vi "drawLabel.vi"(0 "reference":refnum<class "StateTransitionEdge.lvclass">, 1 "graphics":refnum<class "Graphics.lvclass">, 5 "error in (no error)":errorcluster) -> (14 "reference out":refnum<class "StateTransitionEdge.lvclass">, 19 "error out":errorcluster)   [LabVIEW 2012, in "StateTransitionEdge.lvclass"]
doc: "private void drawLabel(Graphics2D g2)"
uses:
  <resource>/Framework/Providers/Open_GDS/UML/StateTransitionEdge_class/StateTransitionEdge.lvclass
  <resource>/Framework/Providers/Open_GDS/UML/Graphics_class/Graphics.lvclass
  <resource>/Framework/Providers/Open_GDS/UML/General/Point/Point Point2D.ctl
  <resource>/Framework/Providers/Open_GDS/UML/SegmentedLineEdge_class/SegmentedLineEdge.lvclass
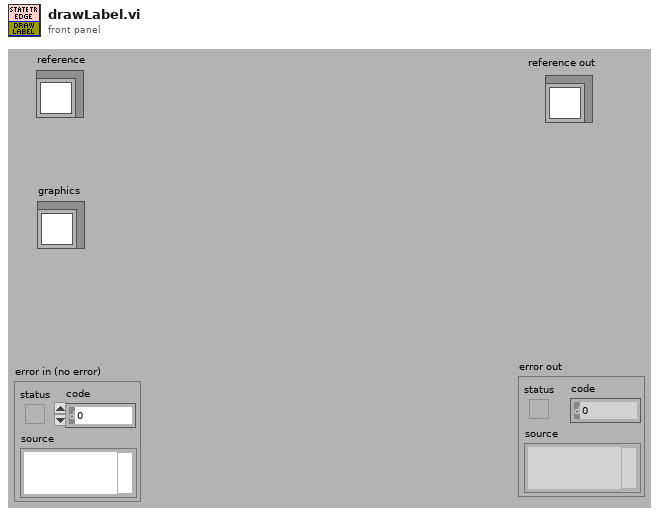
[diagram p1: front panel]
types:
  T1 = typedef "Point Point2D.ctl" = cluster{"x":dbl, "y":dbl}
  T2 = typedef "SegmentedLineEdge.lvclass/ObjectAttributes.ctl" = cluster{"lineStyle":refnum<class "LineStyle.lvclass">, "startArrowHead":refnum<class "ArrowHead.lvclass">, "endArrowHead":refnum<class "ArrowHead.lvclass">, "startLabel":string, "midLabel":string, "endLabel":string, "MidLabelOffset":T1, "SplitWire":bool}
  T3 = typedef "Rectangle Rectangle2D.ctl" = cluster{"x":dbl, "y":dbl, "width":dbl, "height":dbl}
  T4 = cluster{"x":i32, "y":i32, "width":i32, "height":i32}
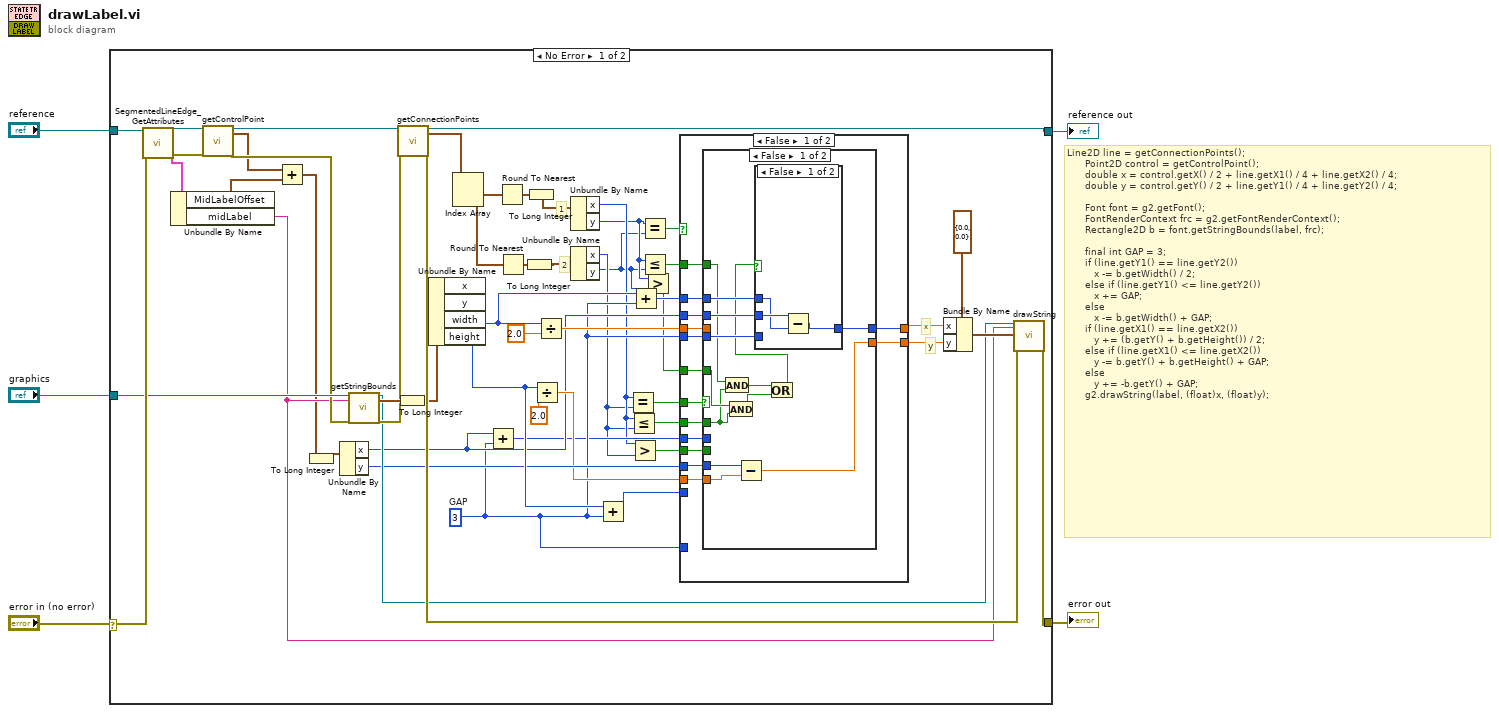
[diagram p0: block diagram]
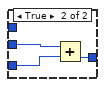
[diagram p2: hidden frame]
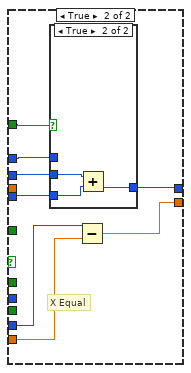
[diagram p3: hidden frame]
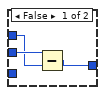
[diagram p4: hidden frame]
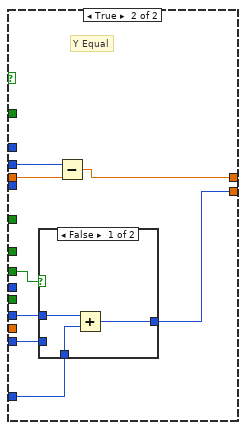
[diagram p5: hidden frame]
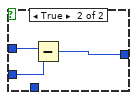
[diagram p6: hidden frame]
diagram:
  # "Line2D line = getConnectionPoints();\n      Point2D control = getControlPoint();\n      double x = control.getX() / 2 + line.getX1() / 4 + line.getX2() / 4;\n      double y = control.getY() / 2 + line.getY1() / 4 + line.getY2() / 4;\n\n      Font font = g2.getFont();\n      FontRenderContext frc = g2.getFontRenderContext();\n      Rectangle2D b = font.getStringBounds(label, frc);      \n\n      final int GAP = 3;\n      if (line.getY1() == line.getY2())\n         x -= b.getWidth() / 2;\n      else if (line.getY1() <= line.getY2())\n         x += GAP;\n      else\n         x -= b.getWidth() + GAP;\n      if (line.getX1() == line.getX2())\n         y += (b.getY() + b.getHeight()) / 2;\n      else if (line.getX1() <= line.getX2())\n         y -= b.getY() + b.getHeight() + GAP;\n      else\n         y += -b.getY() + GAP;\n      g2.drawString(label, (float)x, (float)y);"
  n1 = case shown="No Error" "error in (no error)" {
    selector: "error in (no error)" -> [w57 w120]
    tunnel: "reference" -> [w58 w121]
    tunnel: [w35 w120] -> w4
    tunnel: [w31 w121] -> w3
    tunnel: "graphics" -> [w54 _]
    frame No Error {
      w14 = 3  # GAP
      # "y"
      # "x"
      # "2"
      # "1"
      n2 = call <resource>:"SegmentedLineEdge_GetAttributes.vi"("reference in"=w58, "error in (no error)"=w57) -> ("reference out"=w56:refnum<class "StateTransitionEdge.lvclass">, "Data"=w6:T2, "error out"=w55:errorcluster)  [unwired: 14 in, 1 out]
      n3 = Unbundle By Name(w6) -> ("MidLabelOffset"=w29:T1, "midLabel"=w32:string)
      n4 = call <resource>:"getControlPoint.vi"("reference"=w56, "error in (no error)"=w55) -> ("reference out"=w43:refnum<class "StateTransitionEdge.lvclass">, "point"=w46:T1, "error out"=w53:errorcluster)  [unwired: 15 out]
      n5 = Add(x=w46, y=w29) -> (x+y=w30:T1)
      n6 = To Long Integer(number=w30) -> (32bit integer=w23:cluster{"x":i32, "y":i32})
      n7 = Unbundle By Name(w23) -> ("x"=w15:i32, "y"=w19:i32)
      n8 = call-dynamic "getStringBounds.vi"("reference"=w54, "text"=w32, "error in (no error)"=w53) -> ("reference out"=w33:refnum<class "Graphics.lvclass">, "bounds"=w52:T3, "error out"=w44:errorcluster)  [unwired: 14 in]
      n9 = To Long Integer(number=w52) -> (32bit integer=w24:T4)
      n10 = call-dynamic "getConnectionPoints.vi"("reference"=w43, "error in (no error)"=w44) -> ("reference out"=w31:refnum<class "StateTransitionEdge.lvclass">, "line"=w45:T1[], "error out"=w34:errorcluster)  [unwired: 15 in]
      n11 = Unbundle By Name(w24) -> ("width"=w37:i32, "height"=w22:i32)  [unwired: 2 out]
      n12 = Index Array(array=w45) -> (element #1=w42:T1, element #2=w41:T1)  [unwired: 2 in]
      n13 = Add(x=w15, y=w14) -> (x+y=w13:i32)
      n14 = Round To Nearest(number=w42) -> (nearest integer value=w26:T1)
      n15 = Round To Nearest(number=w41) -> (nearest integer value=w25:T1)
      n16 = To Long Integer(number=w25) -> (32bit integer=w27:cluster{"x":i32, "y":i32})
      n17 = To Long Integer(number=w26) -> (32bit integer=w28:cluster{"x":i32, "y":i32})
      n18 = Divide(x=w22, y=2.0) -> (x/y=w16:dbl)
      n19 = Divide(x=w37, y=2.0) -> (x/y=w40:dbl)
      n20 = Unbundle By Name(w28) -> ("x"=w12:i32, "y"=w10:i32)
      n21 = Unbundle By Name(w27) -> ("x"=w11:i32, "y"=w9:i32)
      n22 = Add(x=w22, y=w14) -> (x+y=w18:i32)
      n23 = Equal?(x=w12, y=w11) -> (x = y?=w17:bool)
      n24 = Less Or Equal?(x=w12, y=w11) -> (x <= y?=w20:bool)
      n25 = Greater?(x=w12, y=w11) -> (0:w7:bool)
      n26 = Add(x=w37, y=w14) -> (x+y=w36:i32)
      n27 = Equal?(x=w10, y=w9) -> (x = y?=w50:bool)
      n28 = Less Or Equal?(x=w10, y=w9) -> (x <= y?=w38:bool)
      n29 = Greater?(x=w10, y=w9) -> (0:w8:bool)
      n30 = case shown="False" w50 {
        tunnel: [w69 w111] -> w48
        tunnel: w15 -> [w71 w113]
        tunnel: w40 -> [w65 w112]
        tunnel: w38 -> [w72 _]
        tunnel: w14 -> [w70 _]
        tunnel: w36 -> [w68 _]
        tunnel: [w66 w107] -> w21
        tunnel: w20 -> [w61 w110]
        tunnel: w19 -> [w64 w109]
        tunnel: w18 -> [_ w108]
        tunnel: w14 -> [_ w106]
        tunnel: w17 -> [w67 _]
        tunnel: w16 -> [w63 _]
        tunnel: w13 -> [w62 _]
        tunnel: w8 -> [w60 _]
        tunnel: w7 -> [w59 _]
        frame False {
          n31 = case shown="False" w67 {
            tunnel: w72 -> [w75 w99]
            tunnel: w71 -> [w85 w94]
            tunnel: w70 -> [w84 w97]
            tunnel: [w83 w96] -> w69
            tunnel: w68 -> [w82 w98]
            tunnel: [w79 w95] -> w66
            tunnel: w65 -> [_ _]
            tunnel: w64 -> [w81 w93]
            tunnel: w63 -> [w80 w92]
            tunnel: w62 -> [_ _]
            tunnel: w61 -> [w73 _]
            tunnel: w60 -> [w74 _]
            tunnel: w59 -> [_ _]
            frame False {
              n32 = And(x=w75, y=w73) -> (x .and. y?=w78:bool)
              n33 = And(x=w74, y=w73) -> (x .and. y?=w77:bool)
              n34 = Subtract(x=w81, y=w80) -> (x-y=w79:dbl)
              n35 = Or(x=w78, y=w77) -> (x .or. y?=w76:bool)
              n36 = case shown="False" w76 {
                tunnel: w85 -> [w88 w91]
                tunnel: w84 -> [_ w90]
                tunnel: [w86 w89] -> w83
                tunnel: w82 -> [w87 _]
                frame False {
                  n37 = Subtract(x=w88, y=w87) -> (x-y=w86:i32)
                }
                frame True {
                  n38 = Add(x=w91, y=w90) -> (x+y=w89:i32)
                }
              }
            }
            frame True {
              # "X Equal"
              n39 = case shown="True" w99 {
                tunnel: w94 -> [w102 w105]
                tunnel: w97 -> [_ w104]
                tunnel: [w100 w103] -> w96
                tunnel: w98 -> [w101 _]
                frame False {
                  n40 = Subtract(x=w102, y=w101) -> (x-y=w100:i32)
                }
                frame True {
                  n41 = Add(x=w105, y=w104) -> (x+y=w103:i32)
                }
              }
              n42 = Subtract(x=w93, y=w92) -> (x-y=w95:dbl)
            }
          }
        }
        frame True {
          # "Y Equal"
          n43 = case shown="False" w110 {
            tunnel: w109 -> [w116 w119]
            tunnel: w108 -> [_ w118]
            tunnel: [w114 w117] -> w107
            tunnel: w106 -> [w115 _]
            frame False {
              n44 = Add(x=w116, y=w115) -> (x+y=w114:i32)
            }
            frame True {
              n45 = Subtract(x=w119, y=w118) -> (x-y=w117:i32)
            }
          }
          n46 = Subtract(x=w113, y=w112) -> (x-y=w111:dbl)
        }
      }
      n47 = Bundle By Name(cluster=T1 {"x"=0.0, "y"=0.0} ("textPos"), "x"=w48, "y"=w21) -> (w47:T1)
      n48 = call-dynamic "drawString.vi"("reference"=w33, "text"=w32, "textPos"=w47, "error in (no error)"=w34) -> ("error out"=w35:errorcluster)  [unwired: 14 in, 1 out]
    }
    frame Error {
    }
  }
  "reference out" <- w3
  "error out" <- w4
